vi "InterTrial.vi"(8 "error in (no error)":errorcluster, 11 "TrialBasedExperiment in":refnum<class "TrialBasedExperiment.lvclass">) -> (0 "error out":errorcluster, 2 "Timeout":dbl, 3 "TrialBasedExperiment out":refnum<class "TrialBasedExperiment.lvclass">)   [LabVIEW 2011, in "TrialBasedExperiment.lvclass"]
uses:
  TrialBasedExperiment.lvclass
  TrialBasedExperiment.lvclass/TrialBasedExperiment.ctl
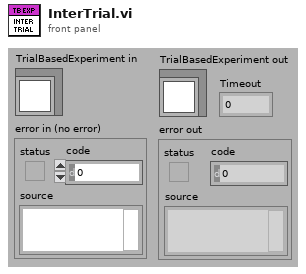
[diagram p1: front panel]
types:
  T1 = enum16{"Get Time", "Get Elapsed Time", "Reset Elapsed Time"}
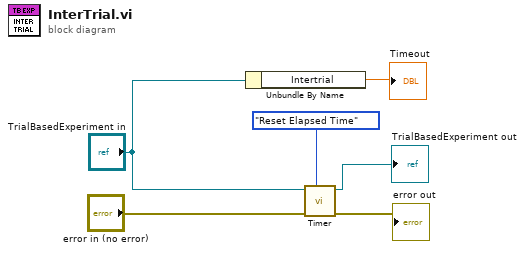
[diagram p0: block diagram]
diagram:
  n1 = Unbundle By Name("TrialBasedExperiment in") -> ("Intertrial"=→"Timeout":dbl)
  n2 = call-dynamic "Timer.vi"("Method"=T1."Reset Elapsed Time", "error in (no error)"="error in (no error)", "BehaviorData in"="TrialBasedExperiment in") -> ("error out"=→"error out":errorcluster, "BehaviorData out"=→"TrialBasedExperiment out":refnum<class "TrialBasedExperiment.lvclass">)  [unwired: 5 in, 2 out]
